vi "Abort.vi"() -> ()   [LabVIEW 2020, in "Setting Lib.lvlib"]
uses:
  Setting Lib.lvlib
  Database Lib.lvlib
panel:
  in  "Restart Software":bool
  out "Error out":errorcluster
  in  "Close Software":bool
  in  "Restart System":bool
  in  "Shut Down System":bool
  out "Error out 2":errorcluster
  in  "Close":bool
  # "Abort"
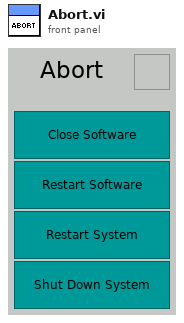
[diagram p1: front panel]
types:
  T1 = cluster{"date/time string":string, "date/time string":string, "code":i32, "date/time string":string, "source":string}
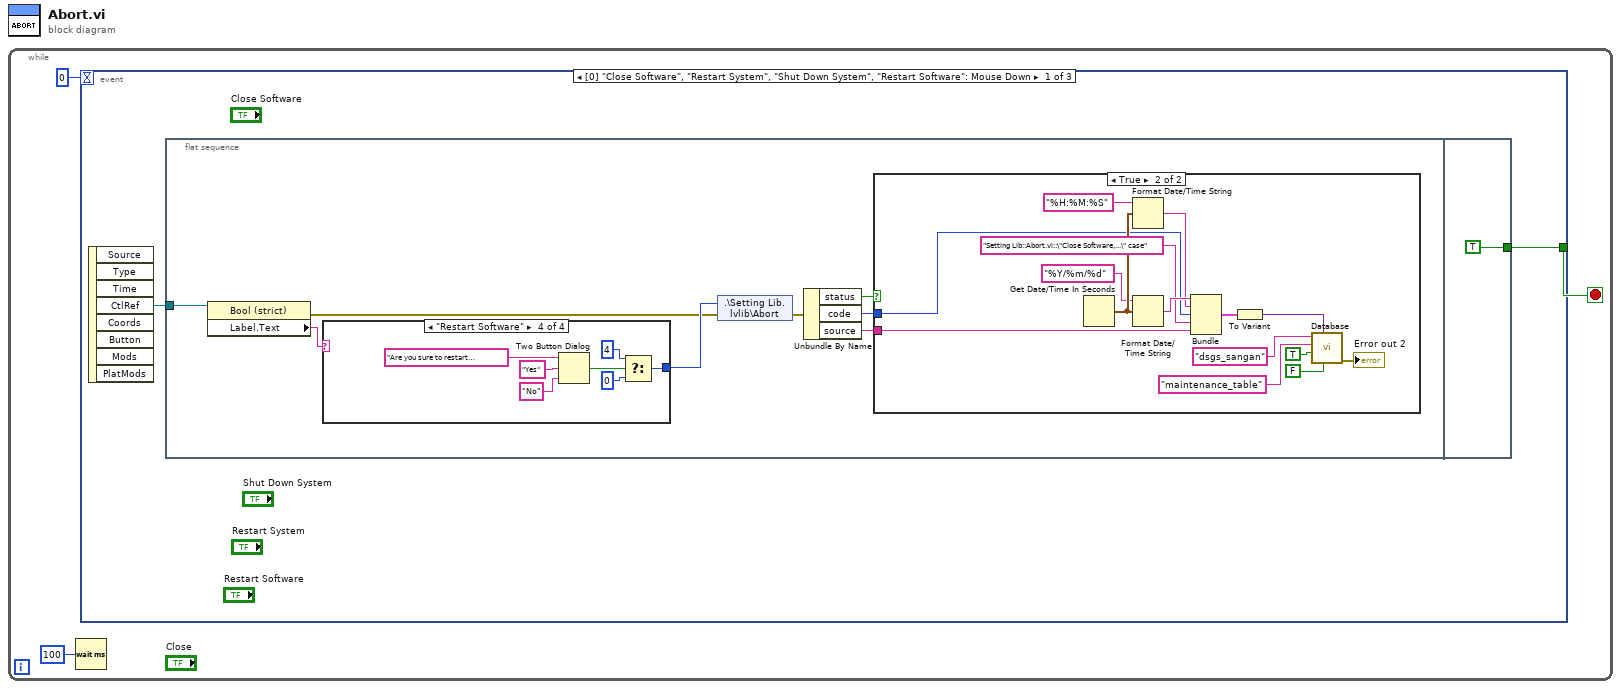
[diagram p0: block diagram]
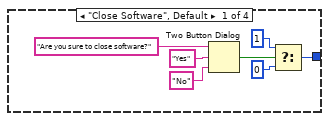
[diagram p3: hidden frame]
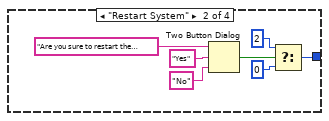
[diagram p4: hidden frame]
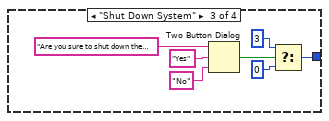
[diagram p5: hidden frame]
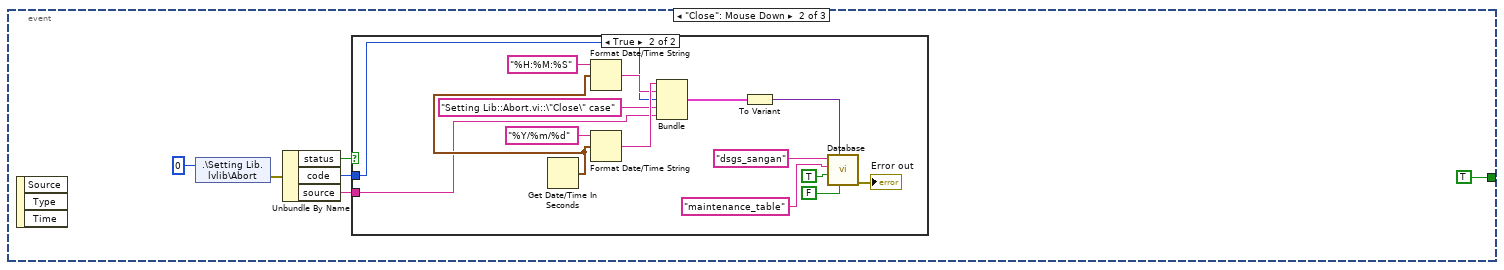
[diagram p6: hidden frame]
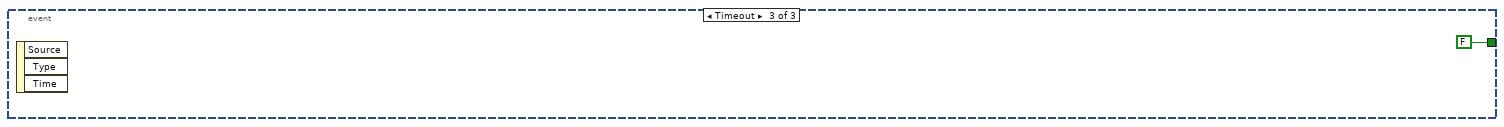
[diagram p8: hidden frame]
diagram:
  n1 = while {
    stop <- w2 stop-if-true
    n2 = Wait (ms)(milliseconds to wait=u32 100) -> ()  [unwired: 1 out]
    n3 = event shown="[0] \"Close Software\", \"Restart System\", \"Shut Down System\", \"Restart Software\": Mouse Down" {
      selector: _ -> [_ _ _]
      dyn-events: _ -> [_ _ _]
      timeout: 0 -> [_ _ _]
      tunnel: [w4 TRUE FALSE] -> w2
      event "Close Software", "Restart System", "Shut Down System", "Restart Software": Mouse Down {
        n4 = event-data() -> ("CtlRef"=w5:refnum<vi>)  [unwired: 1 in, 7 out]
        n5 = flat-sequence {
          tunnel: w5 -> [w13]
          tunnel: [TRUE] -> w4
          frame #0 {
            n6 = property class="Bool (strict)"(reference=w13) -> (error out=w10:errorcluster, "Label.Text"=w12:string)  [unwired: 1 in, 1 out]
            n7 = case shown="\"Restart Software\"" w12 {
              tunnel: [w29 w36 w43 w50] -> w11
              frame "Close Software", Default {
                n8 = Two Button Dialog(message="Are you sure to close software?", 1:"No" ("F button name (\"Cancel\")"), 2:"Yes" ("T button name (\"OK\")")) -> (T button?=w32:bool)
                n9 = Select(t=u8 1, s=w32, f=u8 0) -> (s? t:f=w29:u8)
              }
              frame "Restart System" {
                n10 = Two Button Dialog(message="Are you sure to restart the system?", 1:"No" ("F button name (\"Cancel\")"), 2:"Yes" ("T button name (\"OK\")")) -> (T button?=w39:bool)
                n11 = Select(t=u8 2, s=w39, f=u8 0) -> (s? t:f=w36:u8)
              }
              frame "Shut Down System" {
                n12 = Two Button Dialog(message="Are you sure to shut down the system?", 1:"No" ("F button name (\"Cancel\")"), 2:"Yes" ("T button name (\"OK\")")) -> (T button?=w46:bool)
                n13 = Select(t=u8 3, s=w46, f=u8 0) -> (s? t:f=w43:u8)
              }
              frame "Restart Software" {
                n14 = Two Button Dialog(message="Are you sure to restart software?", 1:"No" ("F button name (\"Cancel\")"), 2:"Yes" ("T button name (\"OK\")")) -> (T button?=w56:bool)
                n15 = Select(t=u8 4, s=w56, f=u8 0) -> (s? t:f=w50:u8)
              }
            }
            n16 = shared-variable ".\\Setting Lib.lvlib\\Abort"(w11, error in=w10) -> (error out=w6:errorcluster)
            n17 = Unbundle By Name(w6) -> ("status"=w8:bool, "code"=w9:i32, "source"=w7:string)
            n18 = case shown="True" w8 {
              tunnel: w9 -> [_ w23]
              tunnel: w7 -> [_ w21]
              frame False {
              }
              frame True {
                n19 = Get Date/Time In Seconds() -> (seconds since 1Jan1904=w28:timestamp)
                n20 = Format Date/Time String(time format string (%c)="%H:%M:%S", seconds (now)=w28) -> (date/time string=w24:string)  [unwired: 1 in]
                n21 = Format Date/Time String(time format string (%c)="%Y/%m/%d", seconds (now)=w28) -> (date/time string=w25:string)  [unwired: 1 in]
                n22 = Bundle("date/time string"=w25, "date/time string"=w24, "code"=w23, "date/time string"="Setting Lib::Abort.vi::\"Close Software,...\" case", "source"=w21) -> (w20:T1)  [unwired: 1 in]
                n23 = To Variant(anything=w20) -> (Variant=w19:variant)
                n24 = call "Database.vi"("Delete row?"=FALSE, "Data"=w19, "Auto Increment ID?"=TRUE, "Table"="maintenance_table", "Connection"="dsgs_sangan") -> ("Error out"=→"Error out 2":errorcluster)  [unwired: 6 in]
              }
            }
          }
          frame #1 {
          }
        }
      }
      event "Close": Mouse Down {
        n25 = event-data() -> ()  [unwired: 1 in, 3 out]
        n26 = shared-variable ".\\Setting Lib.lvlib\\Abort"(u8 0 ("Abort")) -> (error out=w58:errorcluster)  [unwired: 1 in]
        n27 = Unbundle By Name(w58) -> ("status"=w60:bool, "code"=w61:i32, "source"=w59:string)
        n28 = case shown="True" w60 {
          tunnel: w61 -> [_ w73]
          tunnel: w59 -> [_ w71]
          frame False {
          }
          frame True {
            n29 = Get Date/Time In Seconds() -> (seconds since 1Jan1904=w78:timestamp)
            n30 = Format Date/Time String(time format string (%c)="%H:%M:%S", seconds (now)=w78) -> (date/time string=w74:string)  [unwired: 1 in]
            n31 = Format Date/Time String(time format string (%c)="%Y/%m/%d", seconds (now)=w78) -> (date/time string=w75:string)  [unwired: 1 in]
            n32 = Bundle("date/time string"=w75, "date/time string"=w74, "code"=w73, "date/time string"="Setting Lib::Abort.vi::\"Close\" case", "source"=w71) -> (w70:T1)  [unwired: 1 in]
            n33 = To Variant(anything=w70) -> (Variant=w69:variant)
            n34 = call "Database.vi"("Delete row?"=FALSE, "Data"=w69, "Auto Increment ID?"=TRUE, "Table"="maintenance_table", "Connection"="dsgs_sangan") -> ("Error out"=→"Error out":errorcluster)  [unwired: 6 in]
          }
        }
      }
      event Timeout {
        n35 = event-data() -> ()  [unwired: 1 in, 3 out]
      }
    }
  }
